vi "Puff_Stats.vi"(6 "Puff release time (s)":dbl, 8 "Initial Time of Flight":dbl, 10 "Concentrations":dbl[](array[numeric]), 11 "Time (s)":dbl[](array[numeric])) -> (0 "Active Length":i32, 1 "T2 (s)":dbl, 2 "T1 (s)":dbl, 3 "Stats Values":dbl[](array[numeric]), 4 "T1 index":i32)   [LabVIEW 2020]
panel:
  in  "Plot Data":bool
  out "Stats Names":string[](array[string])
  out "Cropped C":dbl[](graph)
  out "Initial":dbl[](graph)
  in  "Factor":dbl=0.7
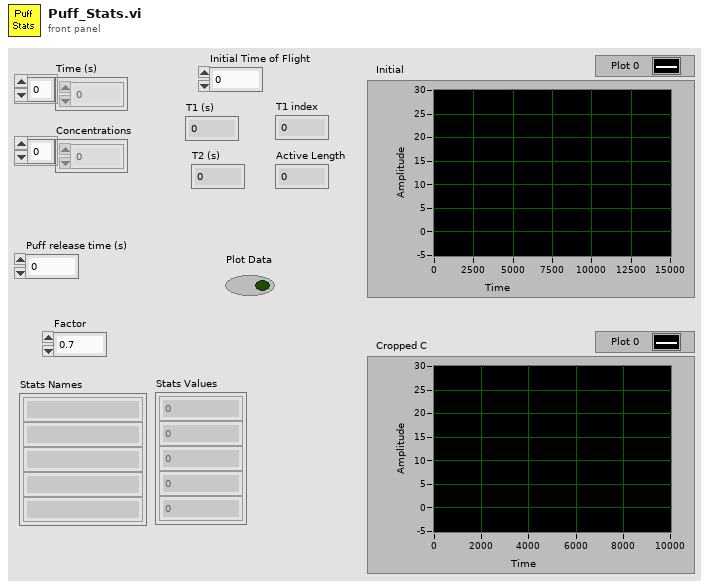
[diagram p1: front panel]
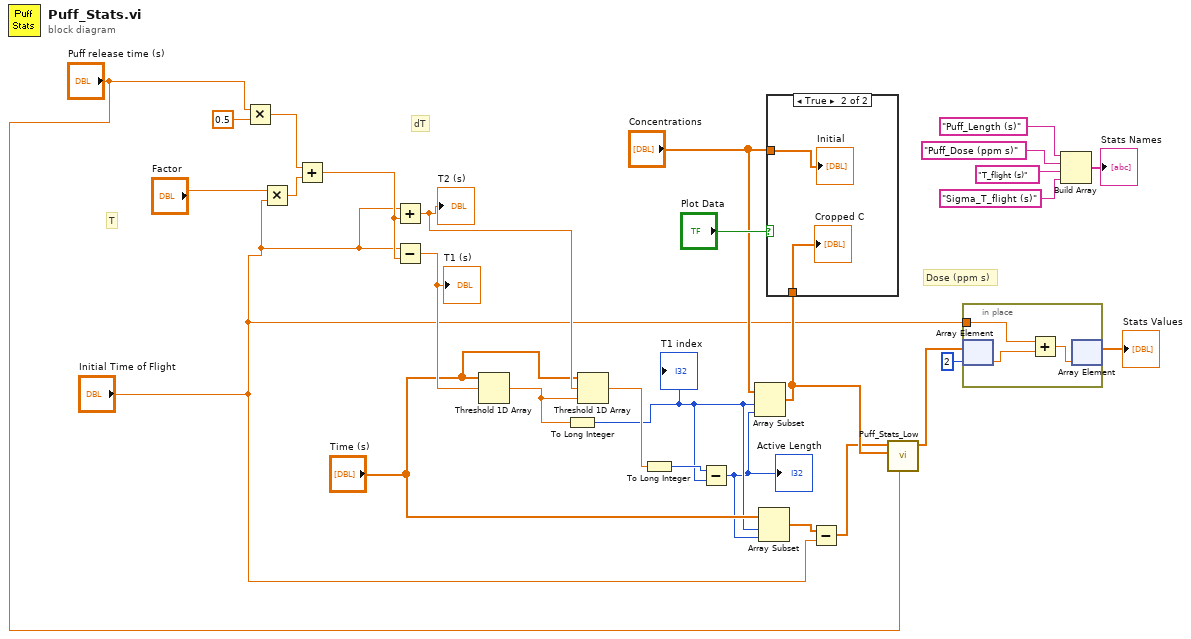
[diagram p0: block diagram]
diagram:
  # "dT"
  # "T"
  # "Dose (ppm s)"
  n1 = Multiply(x="Puff release time (s)", y=0.5) -> (x*y=w27:dbl)
  n2 = Multiply(x="Factor", y="Initial Time of Flight") -> (x*y=w25:dbl)
  n3 = Add(x=w27, y=w25) -> (x+y=w24:dbl)
  n4 = Add(x="Initial Time of Flight", y=w24) -> (x+y=w23:dbl)
  "T2 (s)" <- w23
  n5 = Subtract(x="Initial Time of Flight", y=w24) -> (x-y=w22:dbl)
  "T1 (s)" <- w22
  n6 = Threshold 1D Array(2:w22, 3:"Time (s)") -> (0:w21:dbl)  [unwired: 1 in]
  n7 = To Long Integer(number=w21) -> (32bit integer=w17:i32)
  "T1 index" <- w17
  n8 = Threshold 1D Array(1:w21, 2:w23, 3:"Time (s)") -> (0:w20:dbl)
  n9 = To Long Integer(number=w20) -> (32bit integer=w19:i32)
  n10 = Subtract(x=w19, y=w17) -> (x-y=w16:i32)
  "Active Length" <- w16
  n11 = Array Subset(array="Concentrations", index=w17, length=w16) -> (w7:dbl[])
  n12 = Array Subset(array="Time (s)", index=w17, length=w16) -> (w8:dbl[])
  n13 = case shown="True" "Plot Data" {
    tunnel: w7 -> [_ w30]
    tunnel: "Concentrations" -> [_ w29]
    frame False {
    }
    frame True {
      "Initial" <- w29
      "Cropped C" <- w30
    }
  }
  n14 = Subtract(x=w8, y="Initial Time of Flight") -> (x-y=w3:dbl[])
  n15 = call "Puff_Stats_Low.vi"("Puff release time (s)"="Puff release time (s)", "Concentrations"=w7, "Time (s)"=w3) -> ("Stats"=w6:dbl[])  [unwired: 8 in]
  n16 = in-place {
    in-place-border: "Initial Time of Flight" -> [w32]
    n17 = in-place-array #1(w6, 2) -> (w33:dbl)
    n18 = Add(x=w32, y=w33) -> (x+y=w31:dbl)
    n19 = in-place-array #1(w31) -> (→"Stats Values":dbl[])  [unwired: 1 out]
  }
  n20 = Build Array("Puff_Length (s)", "Puff_Dose (ppm s)", "T_flight (s)", "Sigma_T_flight (s)") -> (→"Stats Names":string[])
